vi "StringJoin.vi"(11 "Array":string[](array[string])) -> (3 "Output":string)   [LabVIEW 2015]
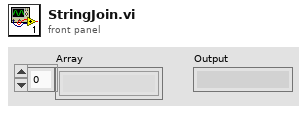
[diagram p1: front panel]
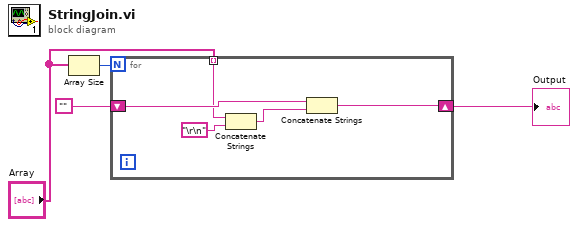
[diagram p0: block diagram]
diagram:
  n1 = Array Size(array="Array") -> (size(s)=w1:i32)
  n2 = for {
    N: w1 -> [_]
    tunnel: "Array" -> [w7] mode=indexing
    shift-right: [w8] -> w3
    shift-left: "" -> [w9]
    n3 = Concatenate Strings(w7, "\r\n") -> (w5:string)
    n4 = Concatenate Strings(w9, w5) -> (w8:string)
  }
  "Output" <- w3
